vi "mod_Message String to Bits.vi"(0 "Message String":string, 5 "bits per symbol":i32, 7 "Preamble/Synchronization":T1={"Sync Number"=59786, "Sync bits"=16, "Sync Start Location, Symbols"=1}, 11 "error in (no error)":errorcluster) -> (4 "output bit stream":i8[](array[numeric]), 6 "Message Length":i32, 15 "error out":errorcluster)   [LabVIEW 2020, in "niDMT.lvlib"]
uses:
  <vilib>/addons/Modulation/niDMT.lvlib
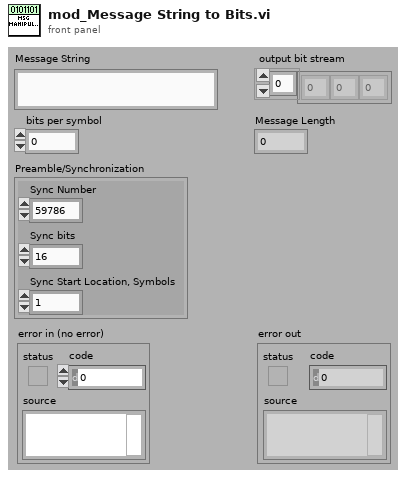
[diagram p1: front panel]
types:
  T1 = cluster{"Sync Number":u32, "Sync bits":i32, "Sync Start Location, Symbols":i32}
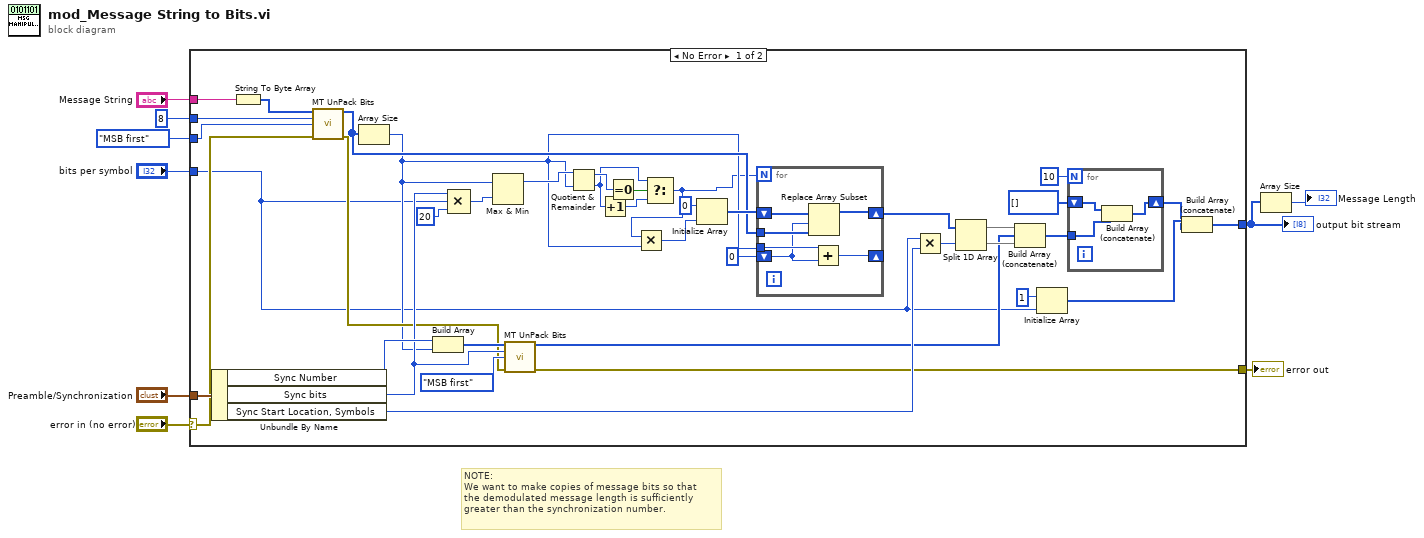
[diagram p0: block diagram]
diagram:
  # "NOTE: \nWe want to make copies of message bits so that \nthe demodulated message length is sufficiently \ngreater than the synchronization number."
  n1 = case shown="No Error" "error in (no error)" {
    selector: "error in (no error)" -> [w19 w59]
    tunnel: "Message String" -> [w49 _]
    tunnel: 8 ("bits per integer") -> [w48 _]
    tunnel: "Preamble/Synchronization" -> [w37 _]
    tunnel: enum16{"MSB first", "LSB first"}."MSB first" ("packed bit order") -> [w20 _]
    tunnel: "bits per symbol" -> [w15 _]
    tunnel: [w24 _] -> w2
    tunnel: [w21 w59] -> w3
    frame No Error {
      n2 = Unbundle By Name(w37) -> ("Sync Number"=w34:u32, "Sync bits"=w32:i32, "Sync Start Location, Symbols"=w30:i32)
      n3 = String To Byte Array(string=w49) -> (unsigned byte array=w36:u8[])
      n4 = call <vilib>:"MT UnPack Bits.vi"("input integers"=w36, "bits per integer"=w48, "packed bit order"=w20, "error in (no error)"=w19) -> ("output bit stream"=w35:i8[], "error out"=w22:errorcluster)  [unwired: 1 in, 9 out]
      n5 = Array Size(array=w35) -> (size(s)=w17:i32)
      n6 = Build Array(w34, w17) -> (w33:u32[])
      n7 = Compound Arithmetic op=MULTIPLY(w32, w15, 20 ("value")) -> (w47:i32)
      n8 = Max & Min(x=w17, y=w47) -> (max(x,y)=w46:i32)  [unwired: 1 out]
      n9 = call <vilib>:"MT UnPack Bits.vi"("input integers"=w33, "bits per integer"=w32, "packed bit order"=enum16{"MSB first", "LSB first"}."MSB first", "error in (no error)"=w22) -> ("output bit stream"=w23:i8[], "error out"=w21:errorcluster)  [unwired: 1 in, 9 out]
      n10 = Quotient & Remainder(x=w46, y=w17) -> (x-y*floor(x/y)=w45:i32, floor(x/y)=w43:i32)
      n11 = Increment(x=w43) -> (x+1=w39:i32)
      n12 = Equal To 0?(x=w45) -> (x = 0?=w44:bool)
      n13 = Select(t=w43, s=w44, f=w39) -> (s? t:f=w10:i32)
      n14 = Multiply(x=w10, y=w17) -> (x*y=w38:i32)
      n15 = Initialize Array(i8 0 ("bits per integer"), w38) -> (w41:i8[])
      n16 = for {
        N: w10 -> [_]
        shift-right: [w53] -> w28
        shift-left: w41 -> [w58]
        tunnel: w35 -> [w57]
        shift-right: [w54] -> _
        shift-left: 0 ("bits per integer") -> [w55]
        tunnel: w17 -> [w56]
        n17 = Replace Array Subset(array=w58, new element=w57, index=w55) -> (w53:i8[])
        n18 = Add(x=w56, y=w55) -> (x+y=w54:i32)
      }
      n19 = Multiply(x=w15, y=w30) -> (x*y=w29:i32)
      n20 = Split 1D Array(array=w28, index=w29) -> (first subarray=w26:i8[], second subarray=w27:i8[])
      n21 = Build Array (concatenate)(w26, w23, w27) -> (w14:i8[])
      n22 = Initialize Array(i8 1, w15) -> (w18:i8[])
      n23 = for {
        N: 10 -> [_]
        shift-right: [w51] -> w12
        shift-left: i8[] [] -> [w50]
        tunnel: w14 -> [w52]
        n24 = Build Array (concatenate)(w50, w52) -> (w51:i8[])
      }
      n25 = Build Array (concatenate)(w18, w12) -> (w24:i8[])
    }
    frame Error {
    }
  }
  "output bit stream" <- w2
  "error out" <- w3
  n26 = Array Size(array=w2) -> (size(s)=→"Message Length":i32)
